vi "getMTData.vi"(11 "MTILC in":refnum<class "MTILC.lvclass">) -> (2 "MTData":T1 {"Responses"."Temperature" items=["OK", "IllegalFunction", "IllegalDataAddress", "IllegalDataValue", "SlaveDeviceFailure", "Acknowledge", "SlaveDeviceBusy", "NegativeAcknowledge", "MemoryParityError", "GatewayPathUnavailable", "GatewayTargetDeviceFailedToRespond"]}, 3 "MTILC out":refnum<class "MTILC.lvclass">)   [LabVIEW 2016, in "RTMTILC.lvlib" / "MTILC.lvclass"]
uses:
  MTILC.lvclass
  DataTypes/MTData.ctl
  DataTypes/MTConstants.ctl
  DataTypes/MTTelemetry.ctl
  DataTypes/MTResponses.ctl
  Common_RT_Modbus/DataTypes/ExceptionCodes.ctl
  DataTypes/MTTimings.ctl
  MTILC.lvclass/MTILC.ctl
  RTMTILC.lvlib
  Common_RT_Modbus/RTModbus.lvlib
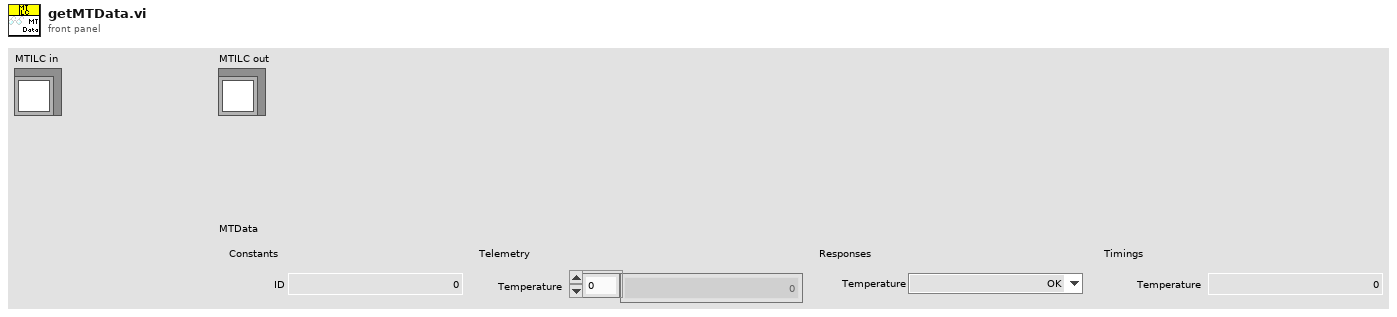
[diagram p1: front panel]
types:
  T1 = typedef "RTMTILC.lvlib/MTData.ctl" = cluster{"Constants":T2, "Telemetry":T3, "Responses":T4, "Timings":T6}
  T2 = typedef "RTMTILC.lvlib/MTConstants.ctl" = cluster{"ID":i16}
  T3 = typedef "RTMTILC.lvlib/MTTelemetry.ctl" = cluster{"Temperature":sgl[]}
  T4 = typedef "RTMTILC.lvlib/MTResponses.ctl" = cluster{"Temperature":T5}
  T5 = typedef "RTModbus.lvlib/ExceptionCodes.ctl" = u16
  T6 = typedef "RTMTILC.lvlib/MTTimings.ctl" = cluster{"Temperature":u32}
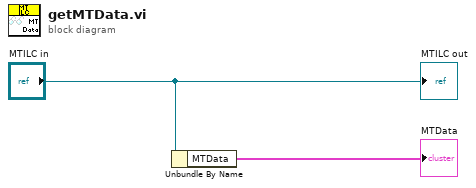
[diagram p0: block diagram]
diagram:
  n1 = Unbundle By Name("MTILC in") -> ("MTData"=→"MTData":T1)
  "MTILC out" <- "MTILC in"
